vi "punto3vero.vi"() -> ()   [LabVIEW 2021]
uses:
  <vilib>/measure/madcrms.llb/Basic Averaged DC-RMS for 1 Chan.vi
  <vilib>/measure/NI_MAPro.lvlib
panel:
  out "Amplitude":dbl
  out "Frequency":dbl
  out "Offset":dbl format="%0.2p"
  out "Acquired signal":dynamicdata(graph)
  out "Generated signal":waveform(dbl)(graph)
  out "Array":dbl[](array[numeric])
  out "Single sample":dynamicdata(graph)
  out "Generator samples chart":dynamicdata(graph)
  in  "Amplitude":dbl=1.0
  in  "Frequency":dbl=1.0
  in  "Offset":dbl
  in  "stop":bool
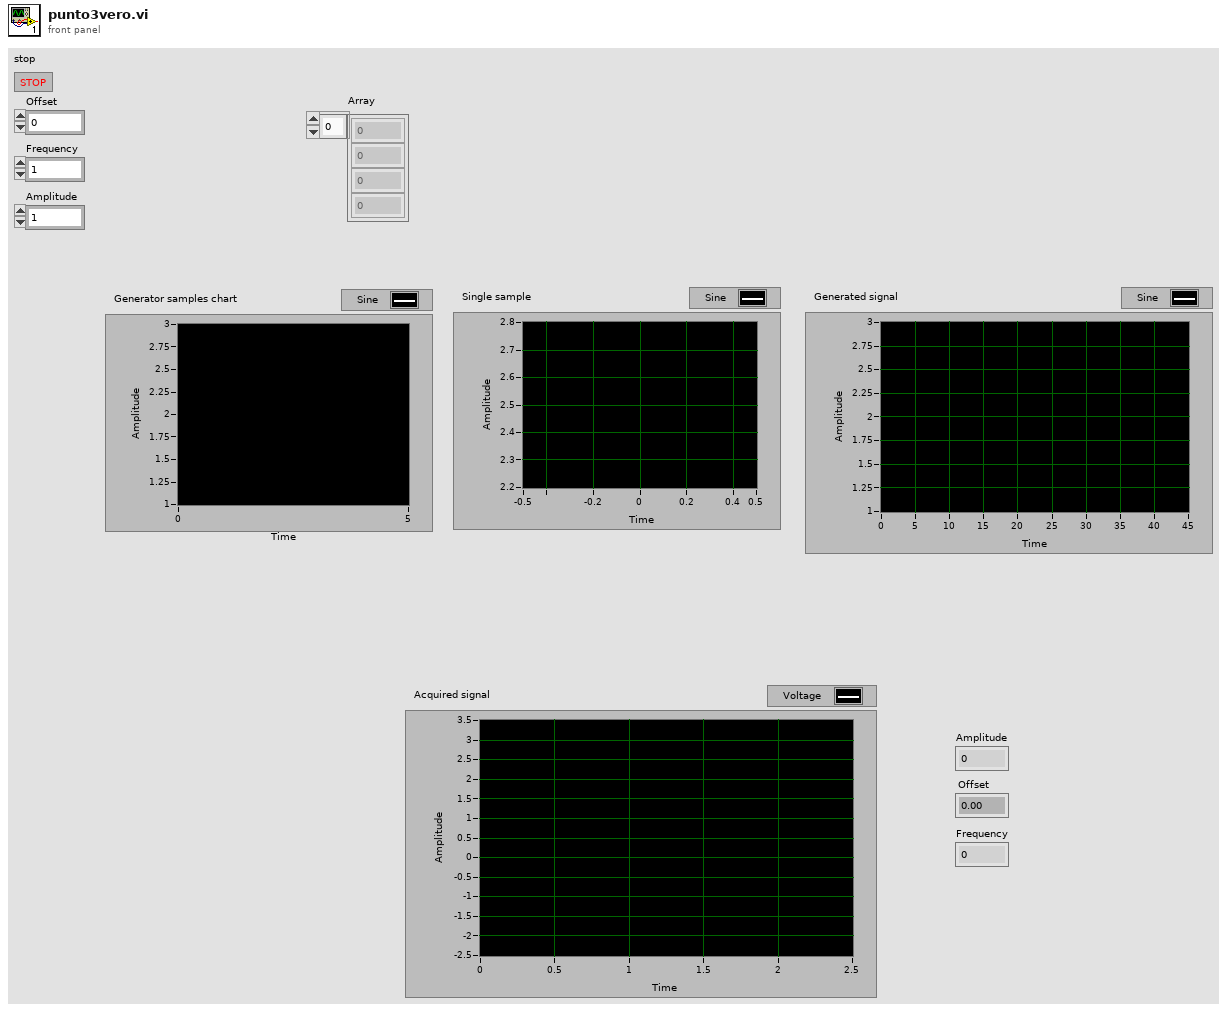
[diagram p1: front panel]
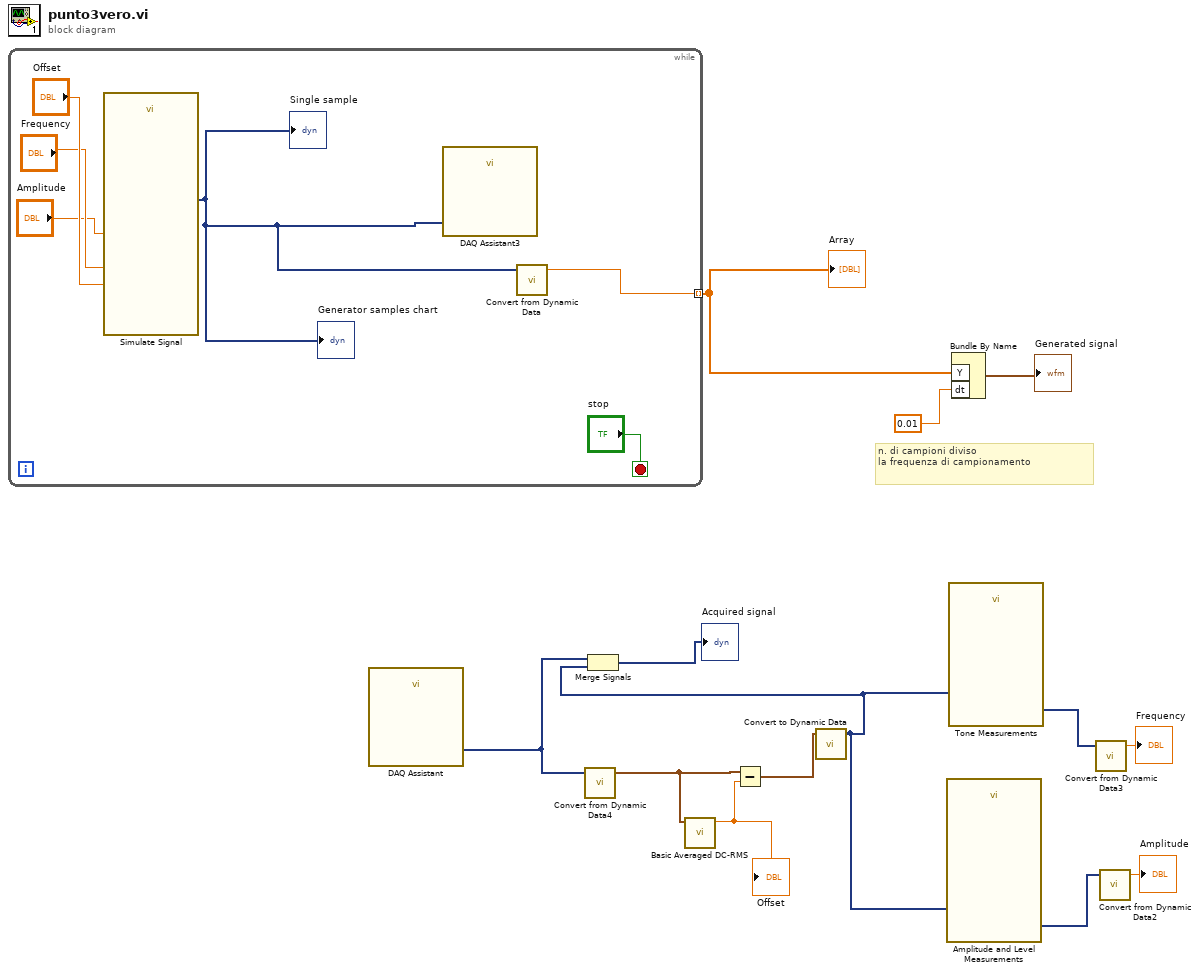
[diagram p0: block diagram]
diagram:
  # "n. di campioni diviso\nla frequenza di campionamento"
  n1 = while {
    tunnel: [w15] -> w11 mode=indexing
    stop <- "stop" stop-if-true
    n2 = call "Simulate Signal"("Offset"="Offset", "Frequency"="Frequency", "Amplitude"="Amplitude") -> ("Sine"=w14:dynamicdata)  [unwired: 11 in, 1 out]
    "Generator samples chart" <- w14
    "Single sample" <- w14
    n3 = call "DAQ Assistant3"("data"=w14) -> ()  [unwired: 17 in, 2 out]
    n4 = call "Convert from Dynamic Data"("Dynamic Data Type"=w14) -> ("Scalar"=w15:dbl)  [unwired: 3 in]
  }
  "Array" <- w11
  n5 = call "DAQ Assistant"() -> ("data"=w1:dynamicdata)  [unwired: 17 in, 2 out]
  n6 = call "Convert from Dynamic Data4"("Dynamic Data Type"=w1) -> ("Waveform"=w9:waveform(dbl))  [unwired: 3 in]
  n7 = call-poly <vilib>:"Basic Averaged DC-RMS.vi"("signal in"=w9) -> ("DC value"=w8:dbl)  [unwired: 7 in, 3 out]
  "Offset" <- w8
  n8 = Subtract(x=w9, y=w8) -> (x-y=w7:waveform(dbl))
  n9 = call "Convert to Dynamic Data"("Waveform"=w7) -> ("Dynamic Data Type"=w2:dynamicdata)  [unwired: 3 in]
  n10 = Merge Signals(w1, w2) -> (→"Acquired signal":dynamicdata)
  n11 = call "Amplitude and Level Measurements"("Signals"=w2) -> ("Peak to Peak"=w6:dynamicdata)  [unwired: 13 in, 1 out]
  n12 = call "Tone Measurements"("Signals"=w2) -> ("Frequency"=w5:dynamicdata)  [unwired: 9 in, 1 out]
  n13 = Bundle By Name("Y"=w11, "dt"=0.01) -> (→"Generated signal":waveform(dbl))  [unwired: 1 in]
  n14 = call "Convert from Dynamic Data3"("Dynamic Data Type"=w5) -> ("Scalar"=→"Frequency":dbl)  [unwired: 3 in]
  n15 = call "Convert from Dynamic Data2"("Dynamic Data Type"=w6) -> ("Scalar"=→"Amplitude":dbl)  [unwired: 3 in]
